vi "calculate_scanner_delays.vi"(8 "error in (no error)":errorcluster, 11 "ScanHeadDL090202 in":refnum<class "ScanHeadDL090202.lvclass">) -> (0 "error out":errorcluster, 3 "ScanHeadDL090202 out":refnum<class "ScanHeadDL090202.lvclass">)   [LabVIEW 2010, in "ScanHeadDL090202.lvclass"]
uses:
  ScanHeadDL090202.lvclass
  Trajectory/GenericTrajectory/GenericTrajectory/GenericTrajectory.lvclass
  common/enumerations/functional_global_action_enum.ctl
  Trajectory/TrajectoryDL091126GenericVoxel/TrajectoryDL091126GenericVoxel/TrajectoryDL091126GenericVoxel.lvclass
  ScanHeadDL090202.lvclass/ScanHeadDL090202.ctl
  common/classes/ErrorController/ErrorController/class_data.vi
  common/classes/ErrorController/ErrorController/ErrorController.lvclass
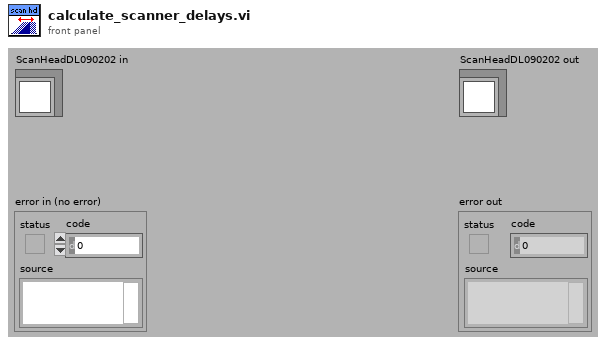
[diagram p1: front panel]
types:
  T1 = typedef "functional_global_action_enum.ctl" = enum16{"get", "set", "reset"}
  T2 = typedef "pixel_raw_data_array.ctl" = dbl[][]
  T3 = typedef "TrajectoryDL091126GenericVoxel.lvclass/transformation_parameters.ctl" = cluster{"scale factor":dbl, "rotation angle":dbl[unit], "tilting angle":dbl[unit], "offset":refnum<class "SpaceVector.lvclass">}
  T4 = cluster{"x":refnum<vi>, "y":refnum<vi>, "z":refnum<vi>}
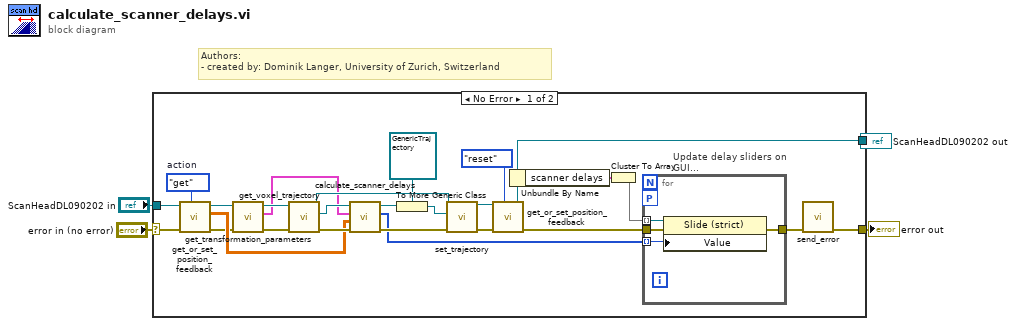
[diagram p0: block diagram]
diagram:
  # "Authors: \n- created by: Dominik Langer, University of Zurich, Switzerland"
  n1 = case shown="No Error" "error in (no error)" {
    selector: "error in (no error)" -> [w27 w36]
    tunnel: [w6 w36] -> w2
    tunnel: "ScanHeadDL090202 in" -> [w28 w35]
    tunnel: [w10 w35] -> w1
    frame No Error {
      w30 = functional_global_action_enum."get"  # action
      n2 = call-dynamic "get_or_set_position_feedback.vi"("action"=w30, "error in (no error)"=w27, "ScanHeadDL090202 in"=w28) -> ("error out"=w16:errorcluster, "position feedback data out"=w25:T2, "ScanHeadDL090202 out"=w13:refnum<class "ScanHeadDL090202.lvclass">)  [unwired: 6 in]
      n3 = call-dynamic "get_transformation_parameters.vi"("error in (no error)"=w16, "ScanHeadDL090202 in"=w13) -> ("error out"=w15:errorcluster, "transformation parameters"=w12:T3, "ScanHeadDL090202 out"=w14:refnum<class "ScanHeadDL090202.lvclass">)  [unwired: 7 in]
      n4 = call-dynamic "get_voxel_trajectory.vi"("error in (no error)"=w15, "ScanHeadDL090202 in"=w14) -> ("error out"=w26:errorcluster, "trajectory"=w24:refnum<class "TrajectoryDL091126GenericVoxel.lvclass">, "ScanHeadDL090202 out"=w21:refnum<class "ScanHeadDL090202.lvclass">)  [unwired: 7 in]
      n5 = call-dynamic "calculate_scanner_delays.vi"("error in (no error)"=w26, "position feedback data"=w25, "transformation parameters"=w12, "TrajectoryDL091126GenericVoxel in"=w24) -> ("error out"=w23:errorcluster, "calculated scanner delays"=w7:i32[], "TrajectoryDL091126GenericVoxel out"=w18:refnum<class "TrajectoryDL091126GenericVoxel.lvclass">)  [unwired: 5 in]
      n6 = To More Generic Class(target class=refnum<class "GenericTrajectory.lvclass"> refnum ("GenericTrajectory.lvclass"), reference=w18) -> (generic class reference=w17:refnum<class "GenericTrajectory.lvclass">)
      n7 = call-dynamic "set_trajectory.vi"("error in (no error)"=w23, "trajectory"=w17, "GenericScanHead.lvclass in"=w21) -> ("error out"=w22:errorcluster, "GenericScanHead.lvclass out"=w20:refnum<class "ScanHeadDL090202.lvclass">)  [unwired: 7 in]
      n8 = call-dynamic "get_or_set_position_feedback.vi"("action"=functional_global_action_enum."reset", "error in (no error)"=w22, "ScanHeadDL090202 in"=w20) -> ("error out"=w11:errorcluster, "ScanHeadDL090202 out"=w10:refnum<class "ScanHeadDL090202.lvclass">)  [unwired: 6 in, 1 out]
      n9 = Unbundle By Name(w10) -> ("scanner delays"=w9:T4)
      n10 = Cluster To Array(cluster=w9) -> (array=w8:refnum<vi>[])
      n11 = for "Update delay sliders on GUI..." {
        tunnel: w11 -> [w34]
        tunnel: [w33] -> w5
        tunnel: w8 -> [w32] mode=indexing
        workers-P: _ -> [_]
        tunnel: w7 -> [w31] mode=indexing
        n12 = property class="Slide (strict)"(reference=w32, error in=w34, "Value"=w31) -> (error out=w33:errorcluster)  [unwired: 1 out]
      }
      n13 = call "send_error.vi"("error in (no error)"=w5) -> ("error out"=w6:errorcluster)  [unwired: 10 in]
    }
    frame Error {
    }
  }
  "error out" <- w2
  "ScanHeadDL090202 out" <- w1
